vi "DN4_AI_OneBufferedRead.vi"(8 "error in (no error)":errorcluster, 11 "Task ID":u32) -> (0 "error out":errorcluster, 2 "data out":dynamicdata(graph), 3 "Task out ID":u32)   [LabVIEW 2009]
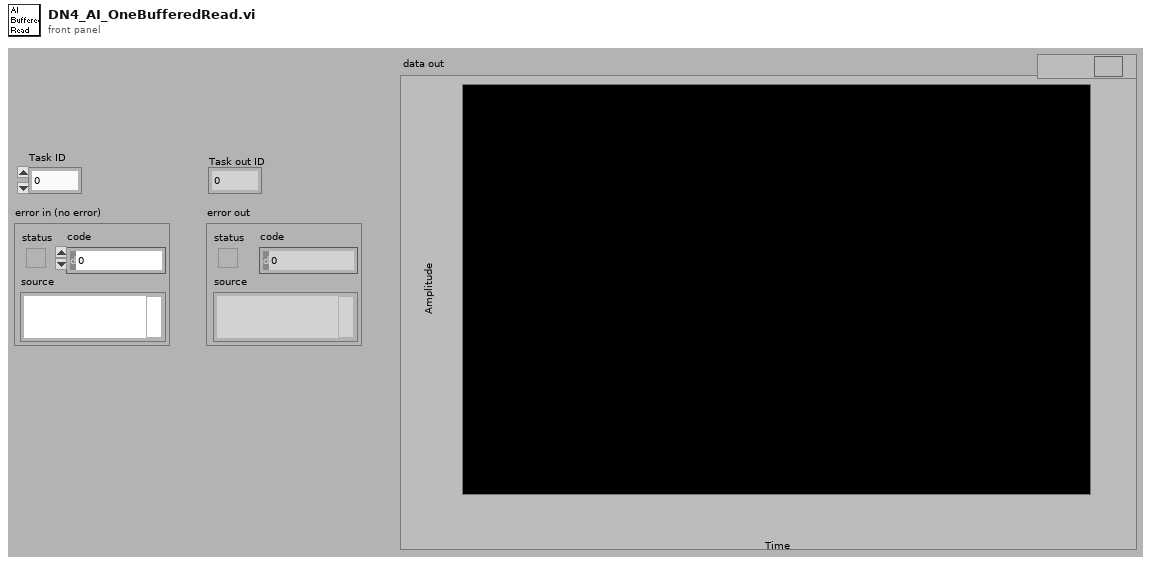
[diagram p1: front panel]
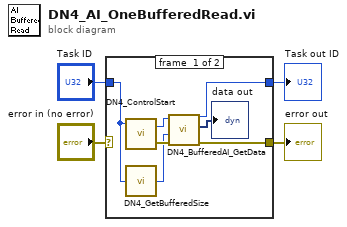
[diagram p0: block diagram]
diagram:
  n1 = case shown="No Error" "error in (no error)" {
    selector: "error in (no error)" -> [_ w13]
    tunnel: [w6 w13] -> w3
    tunnel: "Task ID" -> [w8 w12]
    tunnel: [w5 w12] -> w1
    frame #0 {
      n2 = call <userlib>:"DN4_ControlStart.vi"("Task ID"=w8) -> ("error out"=w11:errorcluster, "Task ID"=w10:u32)  [unwired: 1 in, 1 out]
      n3 = call <userlib>:"DN4_GetBufferedSize.vi"("Task ID"=w8) -> ("return type"=w9:i32)
      n4 = call <userlib>:"DN4_BufferedAI_GetData.vi"("error in (no error)"=w11, "count"=w9, "Task ID"=w10) -> ("error out"=w6:errorcluster, "data out"=→"data out":dynamicdata, "Task ID"=w5:u32)  [unwired: 1 in, 5 out]
    }
    frame #1 {
    }
  }
  "Task out ID" <- w1
  "error out" <- w3
